vi "Set Max values  from distance location.vi"(11 "Vision Data.Vision Distance Center (in)":dbl) -> (3 "output range":cluster{"output high":dbl, "output low":dbl})   [LabVIEW 2017, in "WCDrive2018.lvlib"]
uses:
  WCDrive2018.lvlib
panel:
  out "index of element":i32
  out "What Location Array":bool[](array[boolean])
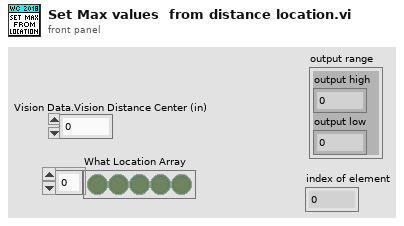
[diagram p1: front panel]
types:
  T1 = enum16{"Unknown", "Close", "Medium-Close", "Medium", "Medium -Far", "Far"}[]
  T2 = enum16{"Unknown", "Close", "Medium-Close", "Medium", "Medium -Far", "Far"}
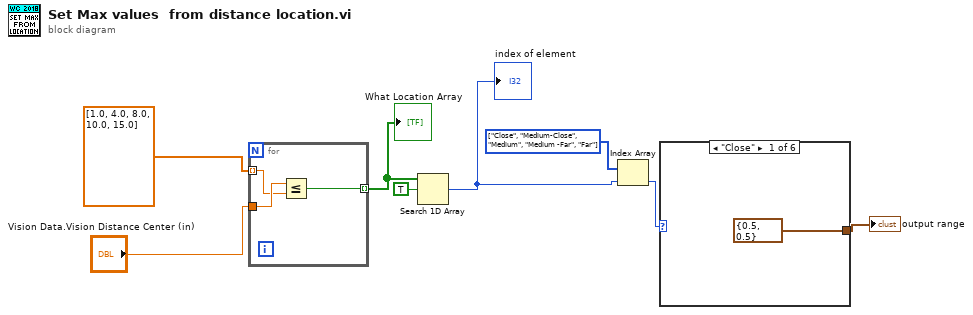
[diagram p0: block diagram]
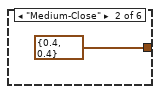
[diagram p2: hidden frame]
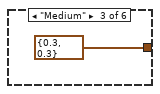
[diagram p3: hidden frame]
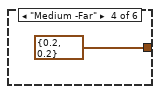
[diagram p4: hidden frame]
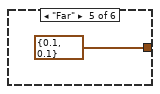
[diagram p5: hidden frame]
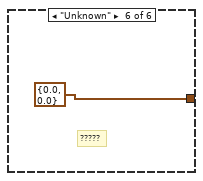
[diagram p6: hidden frame]
diagram:
  w3 = T1 [enum."Close", enum."Medium-Close", enum."Medium", enum."Medium -Far", enum."Far"] items=["Unknown", "Close", "Medium-Close", "Medium", "Medium -Far", "Far"]
  n1 = for {
    tunnel: dbl[] [1.0, 4.0, 8.0, 10.0, 15.0] -> [w10] mode=indexing
    tunnel: "Vision Data.Vision Distance Center (in)" -> [w11]
    tunnel: [w9] -> w5 mode=indexing
    n2 = Less Or Equal?(x=w11, y=w10) -> (x <= y?=w9:bool)
  }
  "What Location Array" <- w5
  n3 = Search 1D Array(1D array=w5, element=TRUE) -> (index of element=w2:i32)  [unwired: 1 in]
  "index of element" <- w2
  n4 = Index Array(array=w3, index=w2) -> (element=w1:T2)
  n5 = case shown="\"Close\"" w1 {
    tunnel: [cluster{"output high":dbl, "output low":dbl} {"output high"=0.5, "output low"=0.5} ("output range") cluster{"output high":dbl, "output low":dbl} {"output high"=0.4, "output low"=0.4} ("output range") cluster{"output high":dbl, "output low":dbl} {"output high"=0.3, "output low"=0.3} ("output range") cluster{"output high":dbl, "output low":dbl} {"output high"=0.2, "output low"=0.2} ("output range") cluster{"output high":dbl, "output low":dbl} {"output high"=0.1, "output low"=0.1} ("output range") cluster{"output high":dbl, "output low":dbl} {"output high"=0.0, "output low"=0.0} ("output range")] -> w8
    frame "Close" {
    }
    frame "Medium-Close" {
    }
    frame "Medium" {
    }
    frame "Medium -Far" {
    }
    frame "Far" {
    }
    frame "Unknown" {
      # "?????"
    }
  }
  "output range" <- w8
